vi "GetErdVersion.vi"(0 "session in":refnum<k35>, 11 "error In":errorcluster) -> (4 "session Out":refnum<k35>, 8 "Erds To Read":string[](array[string]), 15 "error Out":errorcluster)   [LabVIEW 2023]
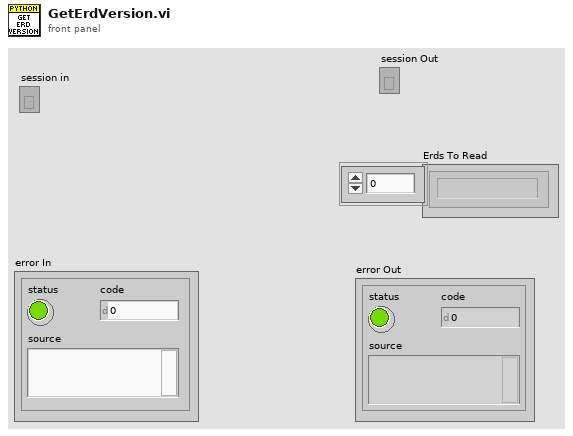
[diagram p1: front panel]
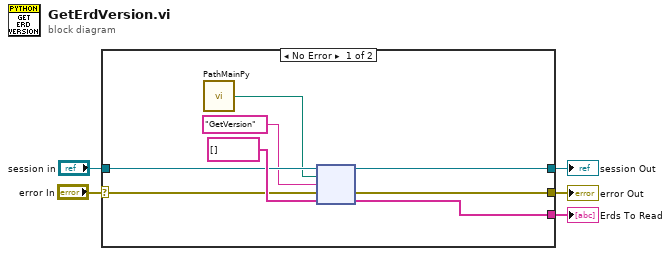
[diagram p0: block diagram]
diagram:
  n1 = case shown="No Error" "error In" {
    selector: "error In" -> [w11 w15]
    tunnel: [w12 _] -> w1
    tunnel: [w9 w15] -> w2
    tunnel: "session in" -> [w10 w14]
    tunnel: [w8 w14] -> w3
    frame No Error {
      n2 = call "PathMainPy.vi"() -> ("path"=w6:path)  [unwired: 15 in]
      n3 = node(w10, w6, "GetVersion" ("function name"), w11, string[] []) -> (w8:refnum<k35>, w9:errorcluster, w12:string[])  [unwired: 2 out]
    }
    frame Error {
    }
  }
  "session Out" <- w3
  "error Out" <- w2
  "Erds To Read" <- w1
